vi "Test MQTT-3.8.4-2.vi"(8 "error in (no error)":errorcluster) -> (0 "error out":errorcluster)   [LabVIEW 2013]
uses:
  source/Control Packets/SUBSCRIBE/Topic Subscription -- cluster.ctl
  source/Control Packets/ControlPacket/QualityOfService -- enum.ctl
  source/Client/Client.lvclass
  <vilib>/addons/_JKI Toolkits/Caraya/classes/Test/Test.lvclass
  source/Control Packets/ControlPacket/ControlPacket.lvclass
  source/Control Packets/SUBSCRIBE/SUBSCRIBE.lvclass
  source/MQTT_Base/MQTT_Base.lvclass
  <vilib>/addons/_JKI Toolkits/Caraya/classes/Assert/Assert.lvclass
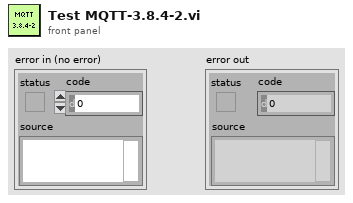
[diagram p1: front panel]
types:
  T1 = typedef "SUBSCRIBE.lvclass/Topic Subscription -- cluster.ctl" = cluster{"Topic Filter":string, "QoS":T2}
  T2 = typedef "ControlPacket.lvclass/QualityOfService -- enum.ctl" = enum16{"0 (At Most Once)", "1 (At Least Once)", "2 (Exactly Once)"}
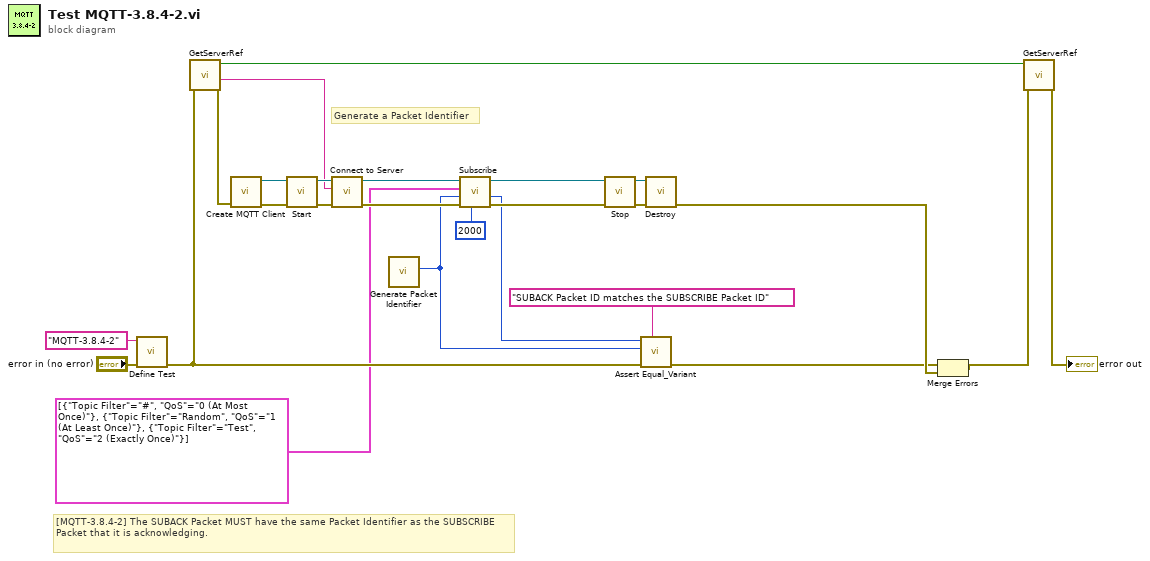
[diagram p0: block diagram]
diagram:
  # "Generate a Packet Identifier"
  # "[MQTT-3.8.4-2] The SUBACK Packet MUST have the same Packet Identifier as the SUBSCRIBE Packet that it is acknowledging."
  n1 = call <vilib>:"Define Test.vi"("error in (no error)"="error in (no error)", "Label (VI Title)"="MQTT-3.8.4-2") -> ("error out"=w7:errorcluster)  [unwired: 9 in]
  n2 = call "GetServerRef.vi"("error in"=w7) -> ("error out"=w22:errorcluster, "Server address"=w1:string, "Created"=w23:bool)  [unwired: 7 in, 1 out]
  n3 = call "Create MQTT Client.vi"("error in (no error)"=w22) -> ("error out"=w11:errorcluster, "Client out"=w12:refnum<class "Client.lvclass">)  [unwired: 9 in]
  n4 = call "Start.vi"("error in (no error)"=w11, "MQTT_Base in"=w12) -> ("error out"=w18:errorcluster, "MQTT_Base out"=w19:refnum<class "Client.lvclass">)  [unwired: 7 in, 1 out]
  n5 = call "Connect to Server.vi"("error in (no error)"=w18, "address (localhost)"=w1, "Client in"=w19) -> ("error out"=w14:errorcluster, "Client out"=w15:refnum<class "Client.lvclass">)  [unwired: 6 in, 1 out]
  n6 = call "Generate Packet Identifier.vi"() -> ("Packet Identifier"=w2:u16)  [unwired: 11 in]
  n7 = call "Subscribe.vi"("timeout (1000 ms)"=2000, "error in (no error)"=w14, "Packet ID (empty: Generate new)"=w2, "Topic Subscriptions"=T1[] [{"Topic Filter"="#", "QoS"=enum."0 (At Most Once)"}, {"Topic Filter"="Random", "QoS"=enum."1 (At Least Once)"}, {"Topic Filter"="Test", "QoS"=enum."2 (Exactly Once)"}], "MQTT_Base in"=w15) -> ("error out"=w9:errorcluster, "SUBACK Packet ID"=w3:u16, "MQTT_Base out"=w10:refnum<class "Client.lvclass">)  [unwired: 3 in, 1 out]
  n8 = call "Stop.vi"("error in (no error)"=w9, "MQTT_Base in"=w10) -> ("error out"=w16:errorcluster, "MQTT_Base out"=w17:refnum<class "Client.lvclass">)  [unwired: 7 in, 1 out]
  n9 = call <vilib>:"Assert Equal_Variant.vi"("Label"="SUBACK Packet ID matches the SUBSCRIBE Packet ID", "error in (no error)"=w7, "Y"=w2, "X"=w3) -> ("error out"=w4:errorcluster)  [unwired: 7 in]
  n10 = call-dynamic "Destroy.vi"("error in (no error)"=w16, "Client in"=w17) -> ("error out"=w5:errorcluster)  [unwired: 8 in, 1 out]
  n11 = Merge Errors(w4, w5) -> (w8:errorcluster)
  n12 = call "GetServerRef.vi"("error in"=w8, "Destroy (F)"=w23) -> ("error out"=→"error out":errorcluster)  [unwired: 6 in, 3 out]
